vi "Sine(SubVI).vi"(4 "error":bool, 5 "stop":bool, 7 "sampling":i32, 8 "length of signal":dbl, 9 "frequency":dbl, 10 "amplitude":dbl, 11 "offset (deg)":dbl) -> (2 "amplitude":dbl[](array[numeric]), 3 "time":dbl[](array[numeric]))   [LabVIEW 2020]
uses:
  <vilib>/numeric/Random Number (Range) DBL.vi
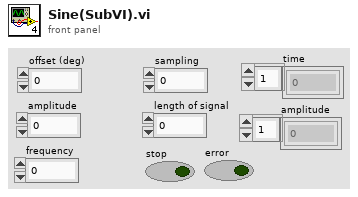
[diagram p1: front panel]
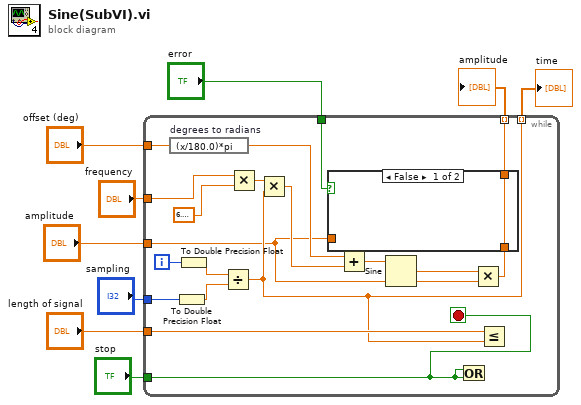
[diagram p0: block diagram]
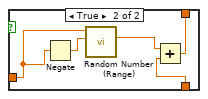
[diagram p2: hidden frame]
diagram:
  n1 = while {
    tunnel: [w13] -> w3 mode=indexing
    tunnel: [w15] -> w2 mode=indexing
    tunnel: "stop" -> [w10]
    tunnel: "length of signal" -> [w17]
    tunnel: "frequency" -> [w22]
    tunnel: "offset (deg)" -> [w19]
    tunnel: "sampling" -> [w21]
    tunnel: "amplitude" -> [w11]
    tunnel: "error" -> [w12]
    i -> [w27]
    stop <- w10 stop-if-true
    n2 = expression code="(x/180.0)*pi" "degrees to radians"(w19) -> (w18:dbl)
    n3 = To Double Precision Float(number=w21) -> (double precision float=w16:dbl)
    n4 = To Double Precision Float(number=w27) -> (double precision float=w25:dbl)
    n5 = Divide(x=w25, y=w16) -> (x/y=w15:dbl)
    n6 = Multiply(x=w22, y=6.283185307179586) -> (x*y=w23:dbl)
    n7 = Multiply(x=w23, y=w15) -> (x*y=w20:dbl)
    n8 = Add(x=w18, y=w20) -> (x+y=w26:dbl)
    n9 = Sine(x=w26) -> (sin(x)=w28:dbl)
    n10 = Or(x=w10, y=w10) -> ()  [unwired: 1 out]
    n11 = Multiply(x=w28, y=w11) -> (x*y=w14:dbl)
    n12 = case shown="False" w12 {
      tunnel: w14 -> [w29 w34]
      tunnel: [w29 w33] -> w13
      tunnel: w11 -> [_ w30]
      frame False {
      }
      frame True {
        n13 = Negate(x=w30) -> (-x=w31:dbl)
        n14 = call-poly <vilib>:"Random Number (Range).vi"("lower bound (0)"=w31, "upper bound (100)"=w30) -> ("number"=w32:dbl)  [unwired: 9 in]
        n15 = Add(x=w32, y=w34) -> (x+y=w33:dbl)
      }
    }
    n16 = Less Or Equal?(x=w17, y=w15) -> ()  [unwired: 1 out]
  }
  "time" <- w2
  "amplitude" <- w3
